vi "Destroy.vi"(0 "reference in":refnum<class "G#SubClass1.lvclass">, 5 "error in (no error)":errorcluster) -> (14 "reference out":refnum<class "G#SubClass1.lvclass">, 19 "error out":errorcluster)   [LabVIEW 2020, in "G#SubClass1.lvclass"]
doc: "Destructor."
uses:
  G#SubClass1.lvclass
  G#BaseClass1_class/G#BaseClass1.lvclass
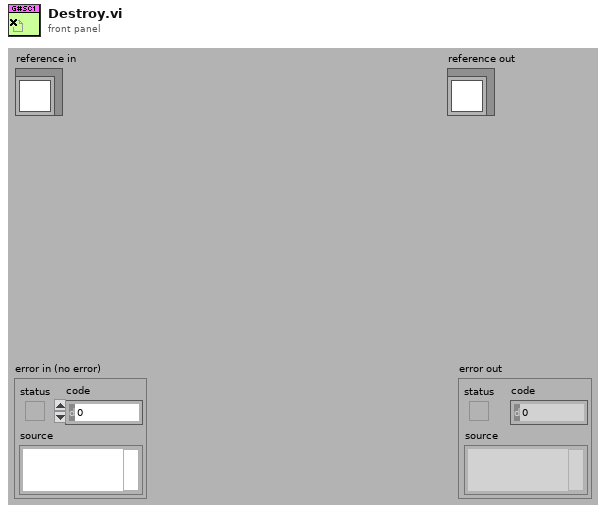
[diagram p1: front panel]
types:
  T1 = typedef "G#SubClass1.lvclass/ObjectAttributes.ctl" = cluster{"SubNumeric":dbl, "TestQueue":refnum<queue>}
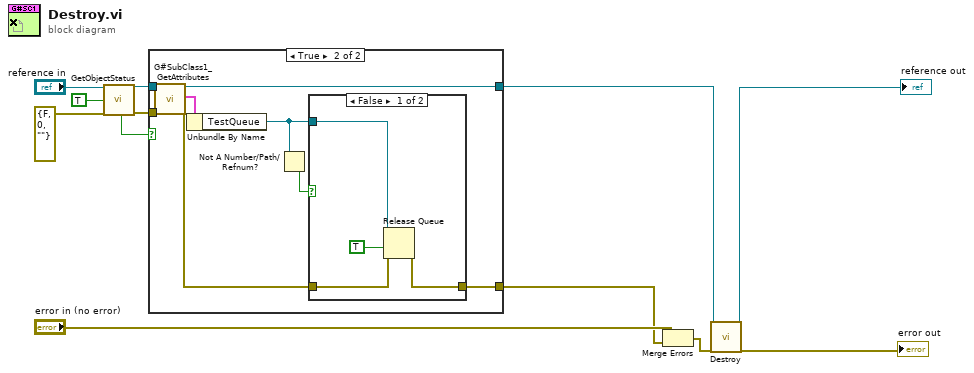
[diagram p0: block diagram]
diagram:
  n1 = call-dynamic "GetObjectStatus.vi"("reference in"="reference in", "simple info (F)"=TRUE ("simple info"), "error in (no error)"=errorcluster {"status"=FALSE, "code"=0, "source"=""}) -> ("last user"=w1:bool, "reference out"=w6:refnum<class "G#SubClass1.lvclass">, "error out"=w7:errorcluster)  [unwired: 5 in, 9 out]
  n2 = case shown="True" w1 {
    tunnel: w7 -> [w13 w22]
    tunnel: w6 -> [w14 w21]
    tunnel: [w14 w20] -> w5
    tunnel: [w13 w17] -> w2
    frame False {
    }
    frame True {
      n3 = call "G#SubClass1_GetAttributes.vi"("reference in"=w21, "error in (no error)"=w22) -> ("reference out"=w20:refnum<class "G#SubClass1.lvclass">, "attributes"=w19:T1, "error out"=w18:errorcluster)  [unwired: 14 in, 1 out]
      n4 = Unbundle By Name(w19) -> ("TestQueue"=w16:refnum<queue>)
      n5 = Not A Number/Path/Refnum?(number/path/refnum=w16) -> (NaN/Path/Refnum?=w15:bool)
      n6 = case shown="False" w15 {
        tunnel: w18 -> [w26 w27]
        tunnel: [w25 w27] -> w17
        tunnel: w16 -> [w23 _]
        frame False {
          n7 = Release Queue(queue=w23, force destroy? (F)=TRUE, error in (no error)=w26) -> (error out=w25:errorcluster)  [unwired: 2 out]
        }
        frame True {
        }
      }
    }
  }
  n8 = Merge Errors("error in (no error)", w2) -> (w11:errorcluster)
  n9 = call-parent "Destroy.vi"("reference in"=w5, "error in (no error)"=w11) -> ("reference out"=→"reference out":refnum<class "G#SubClass1.lvclass">, "error out"=→"error out":errorcluster)  [unwired: 16 in]
